vi "search_mark_place.vi"(9 "square":i32=5, 10 "element":T1=255, 11 "pieceOfWorld in":T2[][](array[typedef])) -> (1 "found?":bool, 2 "column":i32, 3 "row":i32, 5 "volume":i32)   [LabVIEW 2015, in "PolyVIEW.lvclass"]
uses:
  PolyVIEW.lvclass
  actors/world/typedefs/worldCell_cluster.ctl
  actors/world/typedefs/markValue_cluster.ctl
  actors/world/typedefs/markValue.ctl
  actors/world/typedefs/markVolume.ctl
  actors/world/typedefs/amountOfFood.ctl
  actors/world/typedefs/anthillType_enum.ctl
  actors/world/world.lvlib
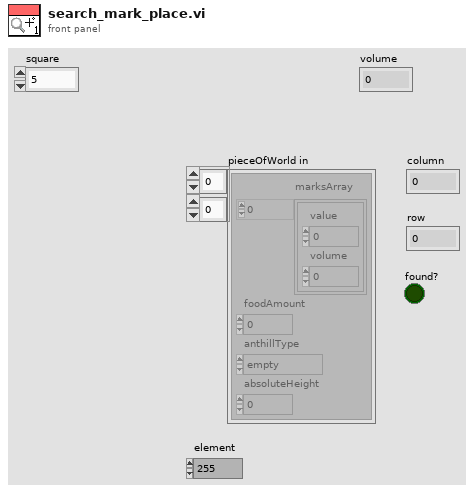
[diagram p1: front panel]
types:
  T1 = typedef "world.lvlib/markValue.ctl" = u8
  T2 = typedef "world.lvlib/worldCell_cluster.ctl" = cluster{"marksArray":T3[], "foodAmount":T5, "anthillType":T6, "absoluteHeight":u8}
  T3 = typedef "world.lvlib/markValue_cluster.ctl" = cluster{"value":T1, "volume":T4}
  T4 = typedef "world.lvlib/markVolume.ctl" = u16
  T5 = typedef "world.lvlib/amountOfFood.ctl" = i32
  T6 = typedef "world.lvlib/anthillType_enum.ctl" = enum16{"empty", "own", "rival"}
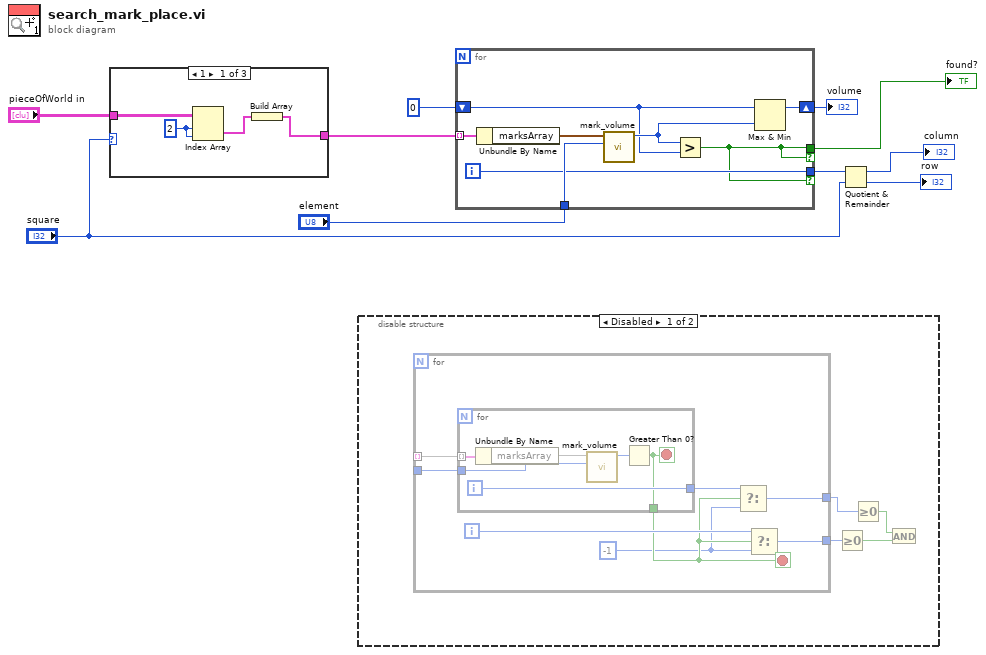
[diagram p0: block diagram]
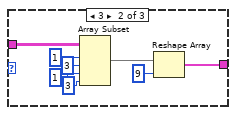
[diagram p2: hidden frame]
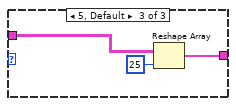
[diagram p3: hidden frame]
diagram:
  n1 = case shown="1" "square" {
    tunnel: "pieceOfWorld in" -> [w14 w20 w23]
    tunnel: [w11 w19 w24] -> w3
    frame 1 {
      w13 = 2 ("index (row)")
      n2 = Index Array(array=w14, index (row)=w13, index (col)=w13) -> (element=w12:T2)
      n3 = Build Array(w12) -> (w11:T2[])
    }
    frame 3 {
      n4 = Array Subset(array=w20, index (row)=1 ("index"), length (row)=3 ("length"), index (col)=1 ("index"), length (col)=3 ("length")) -> (w21:T2[][])
      n5 = Reshape Array(w21, 9 ("dimension size")) -> (w19:T2[])
    }
    frame 5, Default {
      n6 = Reshape Array(w23, 25 ("dimension size")) -> (w24:T2[])
    }
  }
  n7 = disable-structure shown="Disabled" {
    frame Disabled {
      n8 = for {
        tunnel: _ -> [w37] mode=indexing
        tunnel: _ -> [w36]
        tunnel: [w34] -> w27
        tunnel: [w30] -> w26
        i -> [w35]
        stop <- w32 stop-if-true
        w31 = -1
        n9 = for {
          tunnel: w37 -> [w43] mode=indexing
          tunnel: w36 -> [w41]
          tunnel: [w39] -> w33
          tunnel: [w38] -> w32
          i -> [w39]
          stop <- w38 stop-if-true
          n10 = Unbundle By Name(w43) -> ("marksArray"=w42)
          n11 = call "mark_volume.vi"("element"=w41, "marksArray"=w42) -> ("volume"=w40:T4)  [unwired: 9 in]
          n12 = Greater Than 0?(x=w40) -> (x > 0?=w38:bool)
        }
        n13 = Select(t=w33, s=w32, f=w31) -> (s? t:f=w30:i32)
        n14 = Select(t=w35, s=w32, f=w31) -> (s? t:f=w34:i32)
      }
      n15 = Greater Or Equal To 0?(x=w27) -> (x >= 0?=w28:bool)
      n16 = Greater Or Equal To 0?(x=w26) -> (x >= 0?=w29:bool)
      n17 = And(x=w29, y=w28) -> ()  [unwired: 1 out]
    }
    frame Enabled {
    }
  }
  n18 = for {
    tunnel: w3 -> [w51] mode=indexing
    tunnel: "element" -> [w49]
    shift-right: [w46] -> w1
    shift-left: 0 -> [w45]
    tunnel: [w48] -> w9 if=w44
    tunnel: [w44] -> w5 if=w44
    i -> [w48]
    n19 = Unbundle By Name(w51) -> ("marksArray"=w50:T3[])
    n20 = call "mark_volume.vi"("element"=w49, "marksArray"=w50) -> ("volume"=w47:T4)  [unwired: 9 in]
    n21 = Greater?(x=w47, y=w45) -> (0:w44:bool)
    n22 = Max & Min(x=w45, y=w47) -> (max(x,y)=w46:i32)  [unwired: 1 out]
  }
  "found?" <- w5
  "volume" <- w1
  n23 = Quotient & Remainder(x=w9, y="square") -> (x-y*floor(x/y)=→"column":i32, floor(x/y)=→"row":i32)
